vi "ActiView806-Simulator.vi"() -> ()   [LabVIEW 2020]
uses:
  BDF VIs/BDF-Header.ctl
  Sub VIs/AVTCP-FGV Action.ctl
panel:
  out "Played":i32 format="%d s..."
  out "finished":errorcluster
  out "Bytes received":i32
  out "Bytes sent":i32
  in  "Local port":i32=8888
  in  "Play Button":bool
  out "Connected":bool
  out "Listening":bool
  out "Remote port":i32
  out "Remote address":string
  out "Info":string
  in  "BDF file":path
  in  "Cancel Button":bool
  # "Data server"
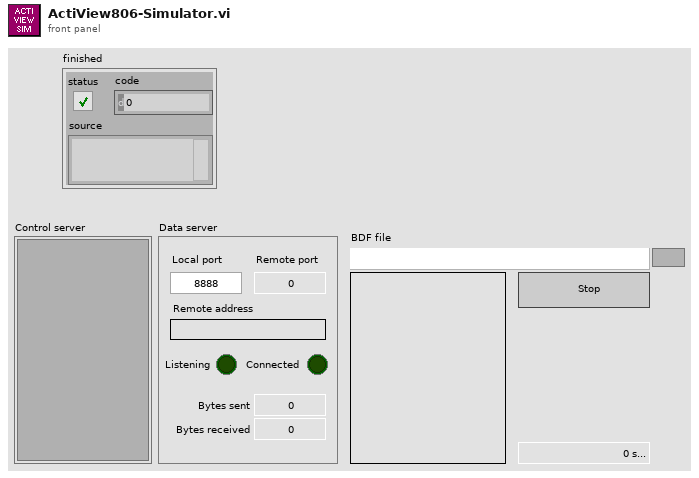
[diagram p1: front panel]
types:
  T1 = typedef "BDF-Header.ctl" = cluster{"ID Code":string, "Local Subject ID":string, "Local Record ID":string, "Date":string, "Time":string, "Header size (bytes)":i32, "Format":string, "Number of records":i32, "Record duration (s)":dbl, "Number of channels":i32, "Labels":string[], "Transducers":string[], "Dimensions":string[], "Physical min":dbl[], "Physical max":dbl[], "Digital min":i32[], "Digital max":i32[], "HP":dbl[], "LP":dbl[], "Samples/record":i32[], "Sample rate":dbl, "Path":path}
  T2 = typedef "AVTCP-FGV Action.ctl" = enum16{"Init", "Write", "Read"}
  T3 = enum8{"Enabled", "Disabled", "Disabled and Grayed Out"}
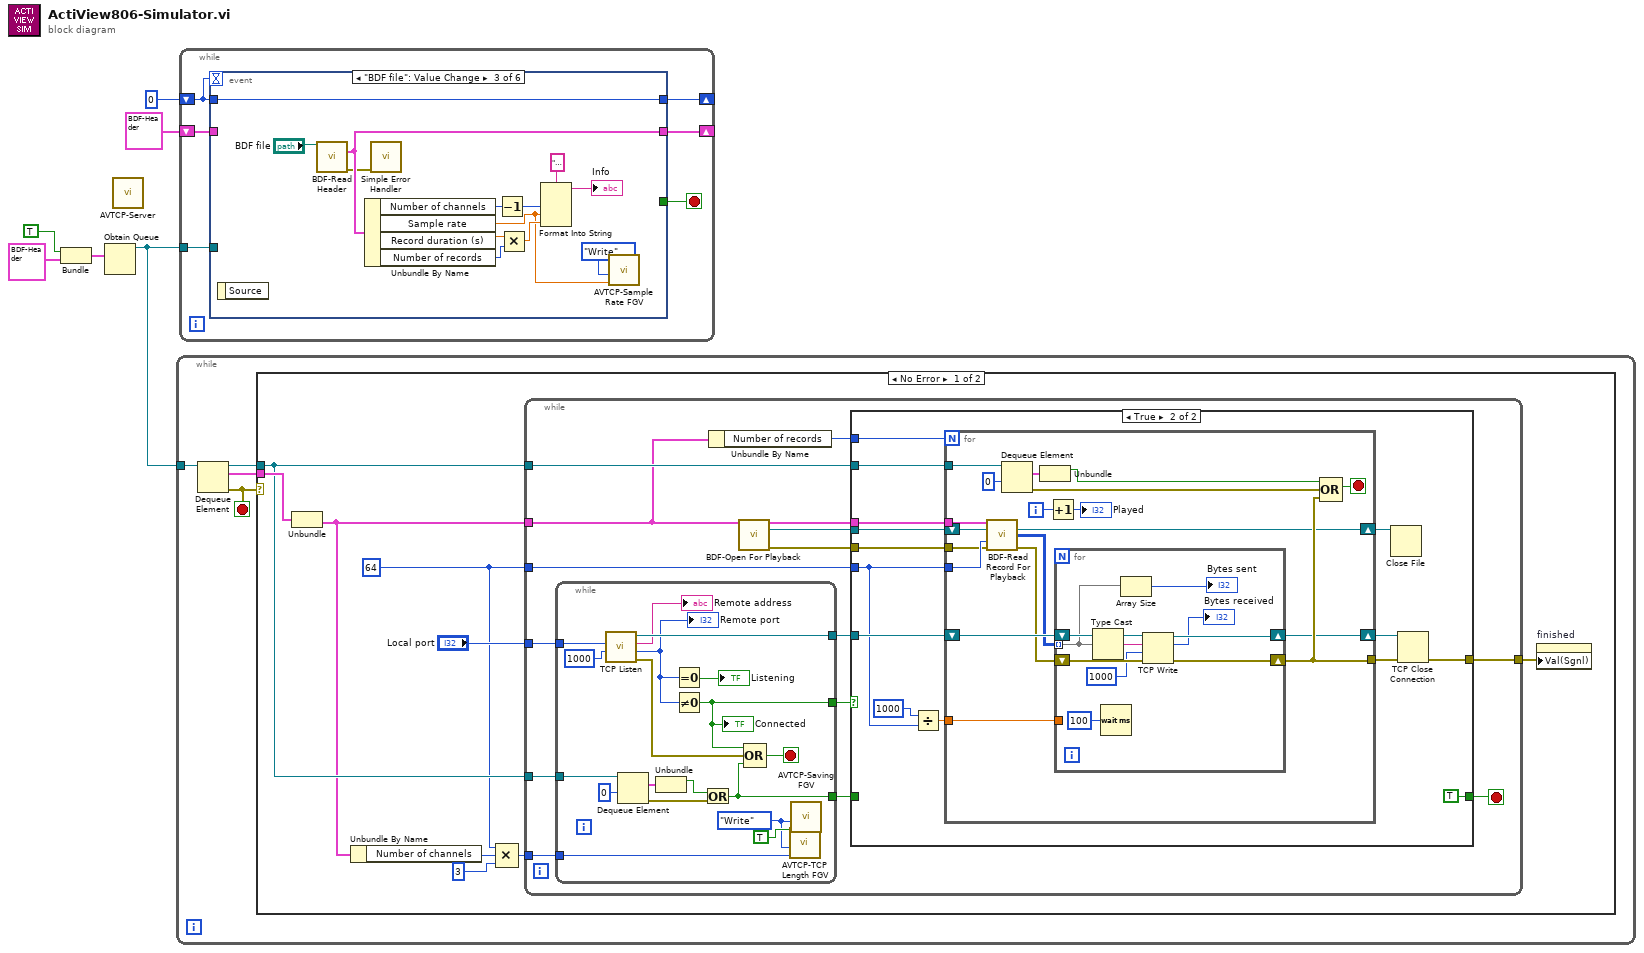
[diagram p0: block diagram]
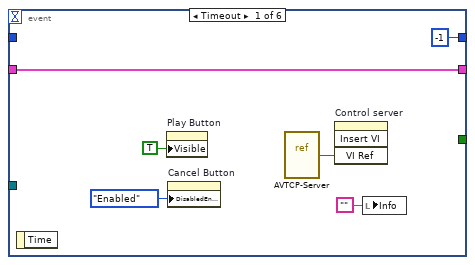
[diagram p4: hidden frame]
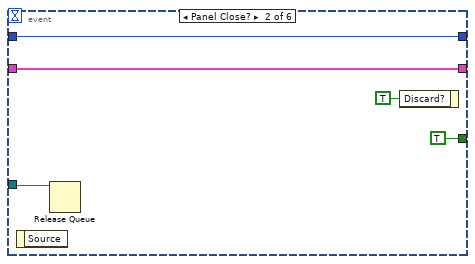
[diagram p5: hidden frame]
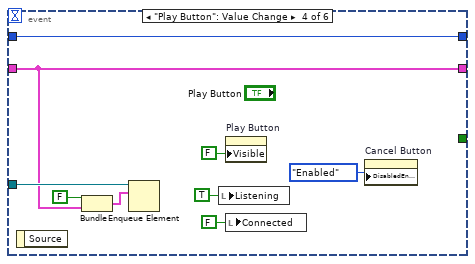
[diagram p6: hidden frame]
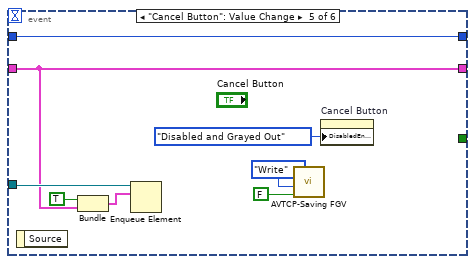
[diagram p7: hidden frame]
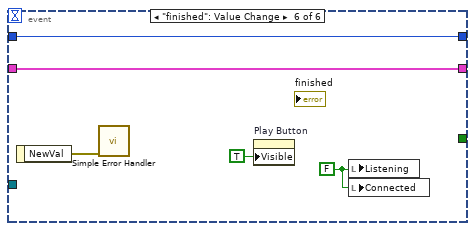
[diagram p8: hidden frame]
diagram:
  n1 = Bundle(TRUE, "Header"=T1 {"ID Code"="", "Local Subject ID"="", "Local Record ID"="", "Date"="", "Time"="", "Header size (bytes)"=0, "Format"="", "Number of records"=0, "Record duration (s)"=0.0, "Number of channels"=0, "Labels"=[], "Transducers"=[], "Dimensions"=[], "Physical min"=[], "Physical max"=[], "Digital min"=[], "Digital max"=[], "HP"=[], "LP"=[], "Samples/record"=[], "Sample rate"=0.0, "Path"=path ""}) -> (w2:cluster{bool, "Header":T1})  [unwired: 1 in]
  n2 = Obtain Queue(element data type=w2) -> (queue out=w1:refnum<queue>)  [unwired: 4 in, 2 out]
  n3 = call "AVTCP-Server.vi"() -> ()  [unwired: 12 in]
  n4 = while {
    tunnel: w1 -> [w10]
    stop <- w7 stop-if-true
    n5 = Dequeue Element(queue=w10) -> (queue out=w8:refnum<queue>, element=w9:cluster{bool, "Header":T1}, error out=w7:errorcluster)  [unwired: 2 in, 1 out]
    n6 = case shown="No Error" w7 {
      tunnel: w9 -> [w19 _]
      tunnel: w8 -> [w17 _]
      frame No Error {
        w11 = 64 ("y")
        n7 = Unbundle(w19) -> ("Header"=w15:T1)  [unwired: 1 out]
        n8 = Unbundle By Name(w15) -> ("Number of channels"=w14:i32)
        n9 = Compound Arithmetic op=MULTIPLY(w11, w14, 3 ("y")) -> (w12:i32)
        n10 = while {
          tunnel: w15 -> [w23]
          tunnel: w17 -> [w34]
          tunnel: "Local port" -> [w33]
          tunnel: [w30] -> w18
          tunnel: w17 -> [w28]
          tunnel: w12 -> [w26]
          tunnel: w11 -> [w24]
          stop <- w29 stop-if-true
          n11 = while {
            tunnel: [w89] -> w27
            tunnel: w34 -> [w95]
            tunnel: [w91] -> w31
            tunnel: w33 -> [w88]
            tunnel: [w82] -> w32
            tunnel: w26 -> [w79]
            stop <- w96 stop-if-true
            w80 = AVTCP-FGV_Action."Write" ("Action")
            n12 = call <vilib>:"TCP Listen.vi"("timeout ms (wait forever: -1)"=1000 ("timeout ms"), "port"=w88) -> ("error out"=w83:errorcluster, "remote port"=w85:u16, "remote address"=→"Remote address":string, "connection ID"=w89:refnum<k5>)  [unwired: 2 in, 4 out]
            "Remote port" <- w85
            n13 = Dequeue Element(queue=w95, timeout in ms (-1)=0) -> (element=w93:cluster{bool, "Header":T1}, error out=w92:errorcluster)  [unwired: 1 in, 2 out]
            n14 = Unbundle(w93) -> (w90:bool)  [unwired: 1 out]
            n15 = Equal To 0?(x=w85) -> (x = 0?=→"Listening":bool)
            n16 = Not Equal To 0?(x=w85) -> (x != 0?=w82:bool)
            "Connected" <- w82
            n17 = Or(x=w90, y=w92) -> (x .or. y?=w91:bool)
            n18 = Compound Arithmetic op=OR(w82, w83, w91) -> (w96:bool)
            n19 = call "AVTCP-TCP Length FGV.vi"("Value in"=w79, "Action"=w80) -> ()  [unwired: 5 in, 1 out]
            n20 = call "AVTCP-Saving FGV.vi"("Value in"=TRUE, "Action"=w80) -> ()  [unwired: 5 in, 1 out]
          }
          n21 = Unbundle By Name(w23) -> ("Number of records"=w25:i32)
          n22 = call "BDF-Open For Playback.vi"("Header"=w23) -> ("Header thru"=w20:T1, "refnum out"=w22:refnum<file>, "error out"=w21:errorcluster)  [unwired: 12 in]
          n23 = case shown="True" w32 {
            tunnel: w31 -> [w35 _]
            tunnel: [_ w44] -> w30
            tunnel: [w35 TRUE] -> w29
            tunnel: w28 -> [_ w48]
            tunnel: w27 -> [_ w47]
            tunnel: w25 -> [_ w43]
            tunnel: w24 -> [_ w40]
            tunnel: w22 -> [_ w39]
            tunnel: w21 -> [_ w38]
            tunnel: w20 -> [_ w37]
            frame False {
            }
            frame True {
              n24 = Divide(x=1000, y=w40) -> (x/y=w41:dbl)
              n25 = for {
                N: w43 -> [_]
                tunnel: w48 -> [w64]
                tunnel: [w59] -> w46
                shift-right: [w58] -> w45
                shift-left: w47 -> [w62]
                tunnel: w41 -> [w57]
                tunnel: w40 -> [w56]
                shift-right: [w53] -> w36
                shift-left: w39 -> [w52]
                tunnel: w38 -> [w51]
                tunnel: w37 -> [w50]
                i -> [w54]
                stop <- w63 stop-if-true
                n26 = call "BDF-Read Record For Playback.vi"("Header"=w50, "refnum in"=w52, "TCP samples"=w56, "error in (no error)"=w51) -> ("refnum out"=w53:refnum<file>, "Array"=w60:u8[][], "error out"=w61:errorcluster)  [unwired: 9 in]
                n27 = Dequeue Element(queue=w64, timeout in ms (-1)=0) -> (element=w67:cluster{bool, "Header":T1}, error out=w66:errorcluster)  [unwired: 1 in, 2 out]
                n28 = Unbundle(w67) -> (w65:bool)  [unwired: 1 out]
                n29 = Increment(x=w54) -> (x+1=→"Played":i32)
                n30 = for {
                  shift-right: [w75] -> w58
                  shift-left: w62 -> [w76]
                  shift-right: [w77] -> w59
                  shift-left: w61 -> [w78]
                  tunnel: w60 -> [w72] mode=indexing
                  tunnel: w57 -> [_]
                  n31 = Type Cast(x=w72) -> (*(type *) &x=w70:string)  [unwired: 1 in]
                  n32 = Wait (ms)(milliseconds to wait=u32 100) -> ()  [unwired: 1 out]
                  n33 = Array Size(array=w72) -> (size(s)=→"Bytes sent":i32)
                  n34 = TCP Write(connection ID=w76, data in=w70, error in (no error)=w78, 9:1000 ("timeout ms (25000)")) -> (connection ID out=w75:refnum<k5>, bytes written=→"Bytes received":i32, error out=w77:errorcluster)
                }
                n35 = Compound Arithmetic op=OR(w65, w66, w59) -> (w63:bool)
              }
              n36 = Close File(refnum=w36) -> ()  [unwired: 1 in, 2 out]
              n37 = TCP Close Connection(connection ID=w45, error in (no error)=w46) -> (error out=w44:errorcluster)  [unwired: 1 in, 1 out]
            }
          }
        }
        n38 = property on="finished" class="Clust (strict)"("Val(Sgnl)"=w18) -> ()  [unwired: 2 in, 2 out]
      }
      frame Error {
      }
    }
  }
  n39 = while {
    shift-right: [w101] -> _
    shift-left: 0 -> [w102]
    shift-right: [w98] -> _
    shift-left: T1 {"ID Code"="", "Local Subject ID"="", "Local Record ID"="", "Date"="", "Time"="", "Header size (bytes)"=0, "Format"="", "Number of records"=0, "Record duration (s)"=0.0, "Number of channels"=0, "Labels"=[], "Transducers"=[], "Dimensions"=[], "Physical min"=[], "Physical max"=[], "Digital min"=[], "Digital max"=[], "HP"=[], "LP"=[], "Samples/record"=[], "Sample rate"=0.0, "Path"=path ""} ("Header") -> [w99]
    tunnel: w1 -> [w97]
    stop <- w100 stop-if-true
    n40 = event shown="[2] \"BDF file\": Value Change" {
      selector: _ -> [_ _ _ _ _ _]
      dyn-events: _ -> [_ _ _ _ _ _]
      timeout: w102 -> [_ _ _ _ _ _]
      tunnel: w102 -> [_ w113 w126 w135 w143 w148]
      tunnel: [-1 w113 w126 w135 w143 w148] -> w101
      tunnel: [_ TRUE _ _ _ _] -> w100
      tunnel: w99 -> [w106 w110 _ w131 w140 w147]
      tunnel: [w106 w110 w124 w131 w140 w147] -> w98
      tunnel: w97 -> [_ w109 _ w132 w141 _]
      event Timeout {
        n41 = event-data() -> ()  [unwired: 1 in, 1 out]
        n42 = property on="Play Button" class="Bool"("Visible"=TRUE) -> ()  [unwired: 2 in, 2 out]
        n43 = property on="Cancel Button" class="Bool"("DisabledEnum"=T3."Enabled" ("Disabled")) -> ()  [unwired: 2 in, 2 out]
        n44 = vi-ref "AVTCP-Server.vi"() -> (w107:refnum<vi>)
        n45 = invoke on="Control server" class="SubPnl" method="Insert VI"("VI Ref"=w107) -> ()  [unwired: 3 in, 4 out]
        n46 = local write "Info"("") -> ()
      }
      event Panel Close? {
        n47 = event-data() -> ()  [unwired: 1 in, 1 out]
        n48 = Release Queue(queue=w109) -> ()  [unwired: 2 in, 3 out]
        n49 = event-data("Discard?"=TRUE) -> ()  [unwired: 1 in, 1 out]
      }
      event "BDF file": Value Change {
        n50 = event-data() -> ()  [unwired: 1 in, 1 out]
        n51 = call "BDF-Read Header.vi"("Path"="BDF file") -> ("Header"=w124:T1, "error out"=w119:errorcluster)  [unwired: 12 in, 1 out]
        n52 = Unbundle By Name(w124) -> ("Number of channels"=w122:i32, "Sample rate"=w115:dbl, "Record duration (s)"=w120:dbl, "Number of records"=w114:i32)
        n53 = call <vilib>:"Simple Error Handler.vi"("error in (no error)"=w119) -> ()  [unwired: 4 in, 5 out]
        n54 = Decrement(x=w122) -> (x-1=w118:i32)
        n55 = Multiply(x=w120, y=w114) -> (x*y=w116:dbl)
        n56 = Format Into String(format string="Channels: %d\nSample rate: %d Hz\nDuration: %#g s", w118, w115, w116) -> (resulting string=→"Info":string)  [unwired: 2 in, 1 out]
        n57 = call "AVTCP-Sample Rate FGV.vi"("Value in"=w115, "Action"=AVTCP-FGV_Action."Write") -> ()  [unwired: 5 in, 1 out]
      }
      event "Play Button": Value Change {
        n58 = event-data() -> ()  [unwired: 1 in, 1 out]
        n59 = Bundle(FALSE, "Header"=w131) -> (w129:cluster{bool, "Header":T1})  [unwired: 1 in]
        n60 = Enqueue Element(queue=w132, element=w129) -> ()  [unwired: 2 in, 3 out]
        n61 = local write "Listening"(TRUE ("Listening")) -> ()
        n62 = property on="Play Button" class="Bool"("Visible"=FALSE) -> ()  [unwired: 2 in, 2 out]
        n63 = local write "Connected"(FALSE ("Connected")) -> ()
        n64 = property on="Cancel Button" class="Bool"("DisabledEnum"=T3."Enabled" ("Disabled")) -> ()  [unwired: 2 in, 2 out]
      }
      event "Cancel Button": Value Change {
        n65 = event-data() -> ()  [unwired: 1 in, 1 out]
        n66 = Bundle(TRUE, "Header"=w140) -> (w139:cluster{bool, "Header":T1})  [unwired: 1 in]
        n67 = Enqueue Element(queue=w141, element=w139) -> ()  [unwired: 2 in, 3 out]
        n68 = call "AVTCP-Saving FGV.vi"("Value in"=FALSE, "Action"=AVTCP-FGV_Action."Write") -> ()  [unwired: 5 in, 1 out]
        n69 = property on="Cancel Button" class="Bool"("DisabledEnum"=T3."Disabled and Grayed Out" ("Disabled")) -> ()  [unwired: 2 in, 2 out]
      }
      event "finished": Value Change {
        w144 = FALSE
        n70 = event-data() -> ("NewVal"=w146:errorcluster)  [unwired: 1 in]
        n71 = call <vilib>:"Simple Error Handler.vi"("error in (no error)"=w146) -> ()  [unwired: 4 in, 5 out]
        n72 = property on="Play Button" class="Bool"("Visible"=TRUE) -> ()  [unwired: 2 in, 2 out]
        n73 = local write "Listening"(w144) -> ()
        n74 = local write "Connected"(w144) -> ()
      }
    }
  }
